vi "Get Number 0.vi"(9 "number 9":string, 10 "number 6":string, 11 "Array":string[][](array[string])) -> (3 "sequence number 0":string)   [LabVIEW 2019, in "Day 8.lvlib"]
uses:
  Day 8.lvlib
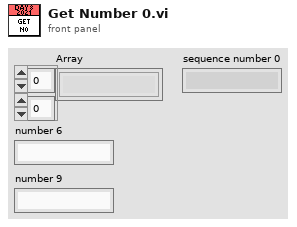
[diagram p1: front panel]
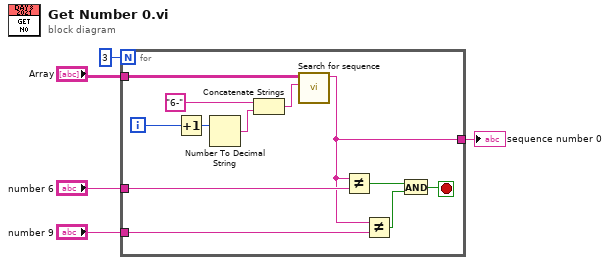
[diagram p0: block diagram]
diagram:
  n1 = for {
    N: 3 -> [_]
    tunnel: "Array" -> [w11]
    tunnel: [w6] -> w4
    tunnel: "number 6" -> [w13]
    tunnel: "number 9" -> [w8]
    i -> [w14]
    stop <- w12 stop-if-true
    n2 = Increment(x=w14) -> (x+1=w15:i32)
    n3 = Number To Decimal String(number=w15) -> (decimal integer string=w16:string)  [unwired: 1 in]
    n4 = Concatenate Strings("6-" ("Pattern For Number Of Letters A"), w16) -> (w10:string)
    n5 = call "Search for sequence.vi"("Pattern For Number Of Letters"=w10, "Array"=w11) -> ("sequence"=w6:string)  [unwired: 9 in]
    n6 = Not Equal?(x=w6, y=w13) -> (x != y?=w9:bool)
    n7 = Not Equal?(x=w6, y=w8) -> (x != y?=w7:bool)
    n8 = And(x=w9, y=w7) -> (x .and. y?=w12:bool)
  }
  "sequence number 0" <- w4
